vi "Climbing.vi"(0 "Start Climb?":bool) -> ()   [LabVIEW 2018]
uses:
  <vilib>/Rock Robotics/WPI/Solenoid/WPI_SolenoidValue.ctl
  <vilib>/Rock Robotics/WPI/Utilities/WPI_GetSetVariantRefNum.vi
  Robot Global Data.vi
  <vilib>/Rock Robotics/WPI/Solenoid/WPI_SolenoidSetEnum.vi
  <vilib>/Rock Robotics/WPI/RobotDrive/WPI_RobotDriveArcadeDrive_Standard(NoSaturation).vi
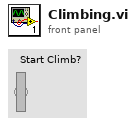
[diagram p1: front panel]
types:
  T1 = typedef "WPI_SolenoidValue.ctl" = enum16{"Off", "On", "Forward", "Reverse"}
  T2 = typedef "WPI_SolenoidDevRef.ctl" = cluster{"DevStatus":errorcluster, "Pneumatics Control Module":u8, "Forward Solenoid Channel":T3, "Reverse Solenoid Channel":T3}
  T3 = typedef "WPI_SolenoidChannel.ctl" = enum8{"Solenoid 0", "Solenoid 1", "Solenoid 2", "Solenoid 3", "Solenoid 4", "Solenoid 5", "Solenoid 6", "Solenoid 7", "Invalid"}
  T4 = typedef "WPI_RobotDriveDevRef.ctl" = cluster{"DevStatus":errorcluster, "Motors[]":T5[], "Square Inputs":bool, "Max Output":dbl}
  T5 = typedef "WPI_MotorControlDeviceRef.ctl" = cluster{"DeviceStatus":errorcluster, "Type":T6, "PWM":cluster{"PWM Channel":T7, "DeadBand":T8}, "CAN":cluster{"Device Number":u8, "SetOutput VI Ref":variant, "GetOutput VI Ref":variant, "Enable VI Ref":variant, "Disable VI Ref":variant, "Data":variant}, "Invert":bool, "DIO PWM":cluster{"PWM \"Enable\" Channel":T7, "DIOChannel":T9, "PWM Rate":dbl}}
  T6 = typedef "WPI_MotorControlType.ctl" = enum16{"PWM", "CAN", "DIO PWM"}
  T7 = typedef "FPGA_DIOPWMChannel.ctl" = enum8{"PWM 0", "PWM 1", "PWM 2", "PWM 3", "PWM 4", "PWM 5", "PWM 6", "PWM 7", "PWM 8", "PWM 9", "PWM MXP 0", "PWM MXP 1", "PWM MXP 2", "PWM MXP 3", "PWM MXP 4", "PWM MXP 5", "PWM MXP 6", "PWM MXP 7", "PWM MXP 8", "PWM MXP 9", "Invalid"}
  T8 = typedef "WPI_PWMDeadband.ctl" = cluster{"Name":string, "maxPositivePwm":i32, "minPositivePwm":i32, "centerPwm":i32, "maxNegativePwm":i32, "minNegativePwm":i32, "angularRange":u16}
  T9 = typedef "FPGA_DIOChannel.ctl" = enum8{"DIO 0", "DIO 1", "DIO 2", "DIO 3", "DIO 4", "DIO 5", "DIO 6", "DIO 7", "DIO 8", "DIO 9", "DIO MXP 0", "DIO MXP 1", "DIO MXP 2", "DIO MXP 3", "DIO MXP 4", "DIO MXP 5", "DIO MXP 6", "DIO MXP 7", "DIO MXP 8", "DIO MXP 9", "DIO MXP 10", "DIO MXP 11", "DIO MXP 12", "DIO MXP 13", "DIO MXP 14", "DIO MXP 15", "SPI Port CS1", "SPI Port CS2", "SPI Port CS3", "SPI Port MISO", "SPI Port MOSI", "Invalid"}
  T10 = typedef "WPI_DigitalInputDevRef.ctl" = cluster{"DevStatus":errorcluster, "DIO Channel":T9}
  T11 = cluster{"X-Axis":dbl, "Y-Axis":dbl, "Z-Axis":dbl}
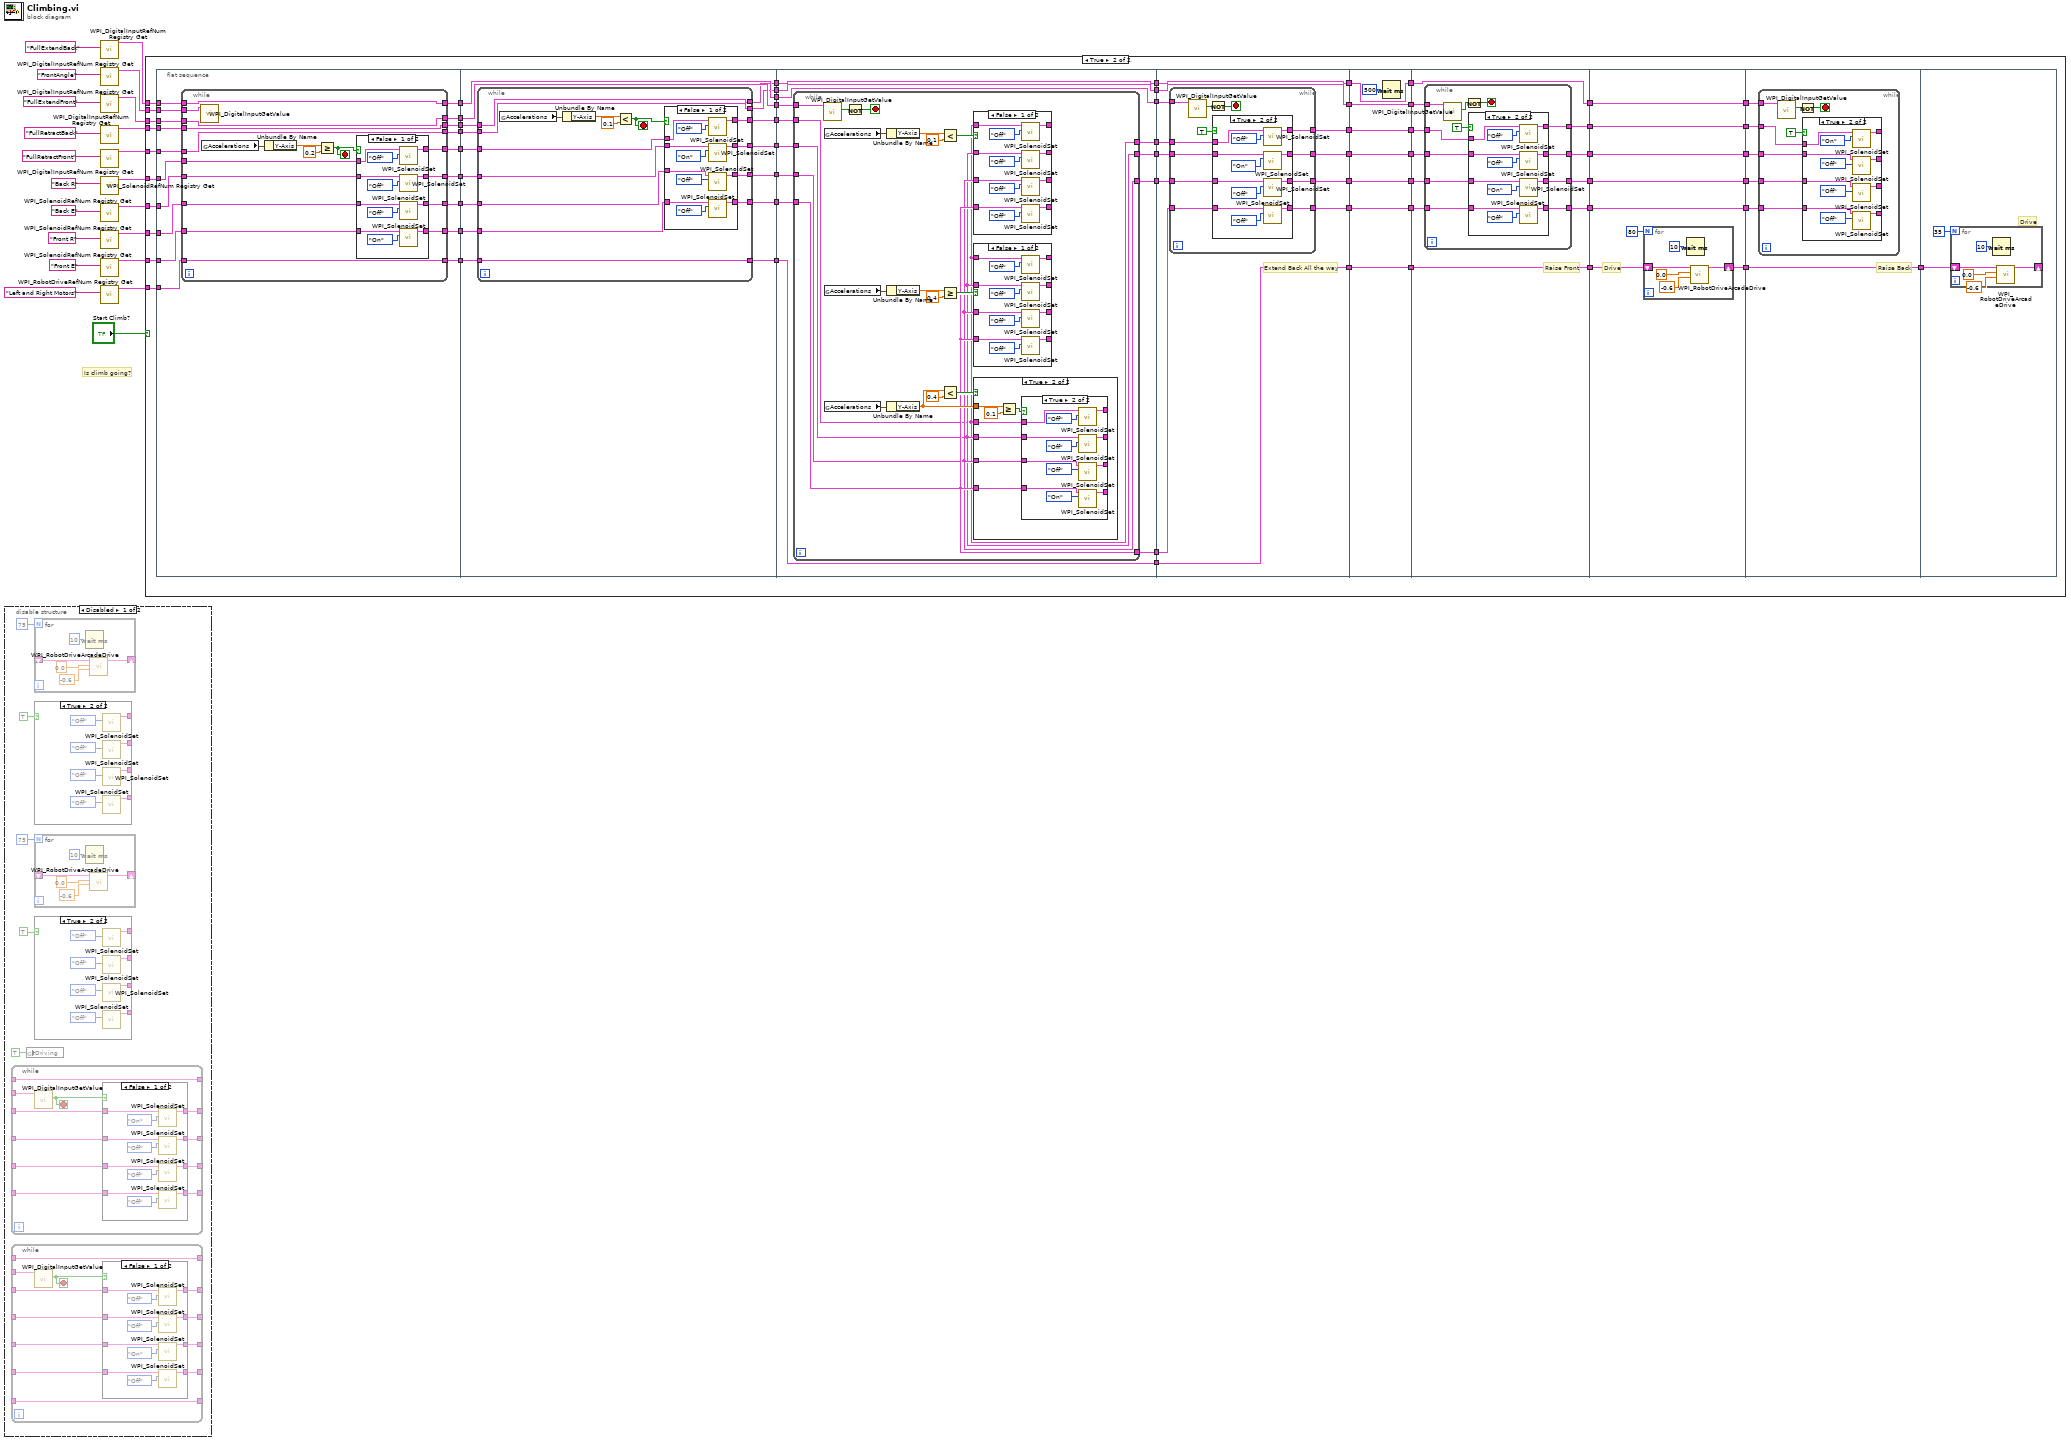
[diagram p0: block diagram]
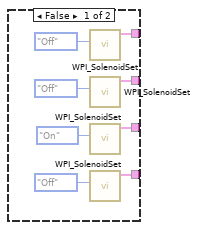
[diagram p2: hidden frame]
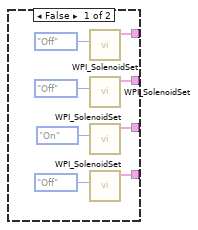
[diagram p3: hidden frame]
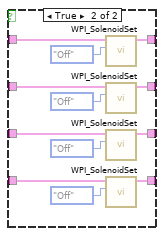
[diagram p4: hidden frame]
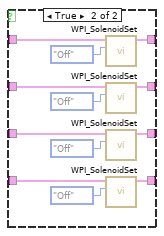
[diagram p5: hidden frame]
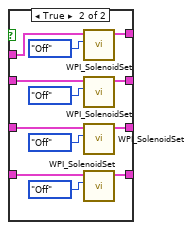
[diagram p8: hidden frame]
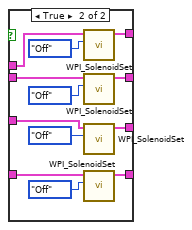
[diagram p9: hidden frame]
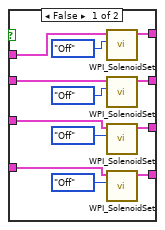
[diagram p11: hidden frame]
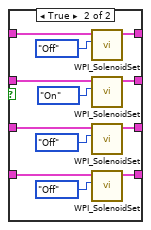
[diagram p12: hidden frame]
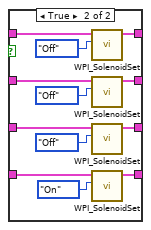
[diagram p13: hidden frame]
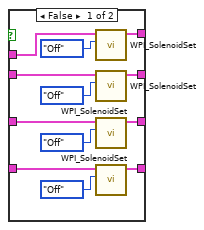
[diagram p14: hidden frame]
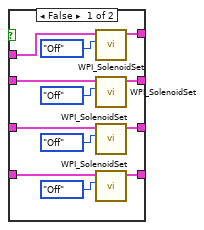
[diagram p15: hidden frame]
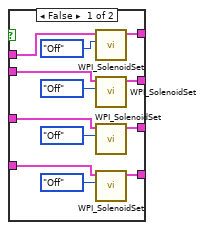
[diagram p16: hidden frame]
diagram:
  # "Is climb going?"
  n1 = disable-structure shown="Disabled" {
    frame Disabled {
      n2 = while {
        tunnel: _ -> [w79]
        tunnel: _ -> [w78]
        tunnel: _ -> [w77]
        tunnel: _ -> [w76]
        tunnel: [w75] -> _
        tunnel: _ -> [w75]
        tunnel: _ -> [w74]
        tunnel: [w72] -> _
        tunnel: [w71] -> _
        tunnel: [w70] -> _
        tunnel: [w69] -> _
        stop <- w73 stop-if-true
        n3 = call <vilib>:"WPI_DigitalInputGetValue.vi"("DigitalInputDevRef"=w74) -> ("Value"=w73:bool)  [unwired: 8 in, 2 out]
        n4 = case shown="False" w73 {
          tunnel: w76 -> [w87 w96]
          tunnel: w77 -> [w86 w97]
          tunnel: w78 -> [w85 w98]
          tunnel: w79 -> [w84 w99]
          tunnel: [w83 w95] -> w69
          tunnel: [w82 w94] -> w70
          tunnel: [w81 w93] -> w71
          tunnel: [w80 w92] -> w72
          frame False {
            n5 = call-poly <vilib>:"WPI_SolenoidSet.vi"("Value"=WPI_SolenoidValue."On", "SolenoidDevRef"=w84) -> ("SolenoidDevRef"=w80:T2)  [unwired: 8 in, 1 out]
            n6 = call-poly <vilib>:"WPI_SolenoidSet.vi"("Value"=WPI_SolenoidValue."Off", "SolenoidDevRef"=w85) -> ("SolenoidDevRef"=w81:T2)  [unwired: 8 in, 1 out]
            n7 = call-poly <vilib>:"WPI_SolenoidSet.vi"("Value"=WPI_SolenoidValue."Off", "SolenoidDevRef"=w86) -> ("SolenoidDevRef"=w82:T2)  [unwired: 8 in, 1 out]
            n8 = call-poly <vilib>:"WPI_SolenoidSet.vi"("Value"=WPI_SolenoidValue."Off", "SolenoidDevRef"=w87) -> ("SolenoidDevRef"=w83:T2)  [unwired: 8 in, 1 out]
          }
          frame True {
            n9 = call-poly <vilib>:"WPI_SolenoidSet.vi"("Value"=WPI_SolenoidValue."Off", "SolenoidDevRef"=w99) -> ("SolenoidDevRef"=w92:T2)  [unwired: 8 in, 1 out]
            n10 = call-poly <vilib>:"WPI_SolenoidSet.vi"("Value"=WPI_SolenoidValue."Off", "SolenoidDevRef"=w98) -> ("SolenoidDevRef"=w93:T2)  [unwired: 8 in, 1 out]
            n11 = call-poly <vilib>:"WPI_SolenoidSet.vi"("Value"=WPI_SolenoidValue."Off", "SolenoidDevRef"=w97) -> ("SolenoidDevRef"=w94:T2)  [unwired: 8 in, 1 out]
            n12 = call-poly <vilib>:"WPI_SolenoidSet.vi"("Value"=WPI_SolenoidValue."Off", "SolenoidDevRef"=w96) -> ("SolenoidDevRef"=w95:T2)  [unwired: 8 in, 1 out]
          }
        }
      }
      n13 = while {
        tunnel: _ -> [w115]
        tunnel: _ -> [w114]
        tunnel: _ -> [w113]
        tunnel: _ -> [w112]
        tunnel: _ -> [w111]
        tunnel: [w110] -> _
        tunnel: _ -> [w110]
        tunnel: [w109] -> _
        tunnel: _ -> [w109]
        tunnel: [w108] -> _
        tunnel: [w107] -> _
        tunnel: [w106] -> _
        tunnel: [w105] -> _
        stop <- w104 stop-if-true
        n14 = call <vilib>:"WPI_DigitalInputGetValue.vi"("DigitalInputDevRef"=w111) -> ("Value"=w104:bool)  [unwired: 8 in, 2 out]
        n15 = case shown="False" w104 {
          tunnel: w115 -> [w123 w132]
          tunnel: w114 -> [w122 w133]
          tunnel: w113 -> [w121 w134]
          tunnel: w112 -> [w120 w135]
          tunnel: [w119 w131] -> w105
          tunnel: [w118 w130] -> w106
          tunnel: [w117 w129] -> w107
          tunnel: [w116 w128] -> w108
          frame False {
            n16 = call-poly <vilib>:"WPI_SolenoidSet.vi"("Value"=WPI_SolenoidValue."Off", "SolenoidDevRef"=w120) -> ("SolenoidDevRef"=w116:T2)  [unwired: 8 in, 1 out]
            n17 = call-poly <vilib>:"WPI_SolenoidSet.vi"("Value"=WPI_SolenoidValue."Off", "SolenoidDevRef"=w121) -> ("SolenoidDevRef"=w117:T2)  [unwired: 8 in, 1 out]
            n18 = call-poly <vilib>:"WPI_SolenoidSet.vi"("Value"=WPI_SolenoidValue."On", "SolenoidDevRef"=w122) -> ("SolenoidDevRef"=w118:T2)  [unwired: 8 in, 1 out]
            n19 = call-poly <vilib>:"WPI_SolenoidSet.vi"("Value"=WPI_SolenoidValue."Off", "SolenoidDevRef"=w123) -> ("SolenoidDevRef"=w119:T2)  [unwired: 8 in, 1 out]
          }
          frame True {
            n20 = call-poly <vilib>:"WPI_SolenoidSet.vi"("Value"=WPI_SolenoidValue."Off", "SolenoidDevRef"=w135) -> ("SolenoidDevRef"=w128:T2)  [unwired: 8 in, 1 out]
            n21 = call-poly <vilib>:"WPI_SolenoidSet.vi"("Value"=WPI_SolenoidValue."Off", "SolenoidDevRef"=w134) -> ("SolenoidDevRef"=w129:T2)  [unwired: 8 in, 1 out]
            n22 = call-poly <vilib>:"WPI_SolenoidSet.vi"("Value"=WPI_SolenoidValue."Off", "SolenoidDevRef"=w133) -> ("SolenoidDevRef"=w130:T2)  [unwired: 8 in, 1 out]
            n23 = call-poly <vilib>:"WPI_SolenoidSet.vi"("Value"=WPI_SolenoidValue."Off", "SolenoidDevRef"=w132) -> ("SolenoidDevRef"=w131:T2)  [unwired: 8 in, 1 out]
          }
        }
      }
      n24 = global write "Robot Global Data.vi" "Driving"(TRUE ("Enable Vision")) -> ()
      n25 = for {
        N: 75 -> [_]
        shift-right: [w47] -> _
        shift-left: _ -> [w46]
        n26 = Wait (ms)(milliseconds to wait=u32 10) -> ()  [unwired: 1 out]
        n27 = call-poly <vilib>:"WPI_RobotDriveArcadeDrive.vi"("Y axis value"=-0.6, "X axis value"=0.0, "RobotDriveDevRef"=w46) -> ("RobotDriveDevRef"=w47:T4)  [unwired: 6 in, 2 out]
      }
      n28 = case shown="True" TRUE {
        tunnel: [w30 w38] -> _
        tunnel: [w29 w37] -> _
        tunnel: [w28 w36] -> _
        tunnel: [w27 w35] -> _
        frame False {
          n29 = call-poly <vilib>:"WPI_SolenoidSet.vi"("Value"=WPI_SolenoidValue."Off") -> ("SolenoidDevRef"=w27:T2)  [unwired: 9 in, 1 out]
          n30 = call-poly <vilib>:"WPI_SolenoidSet.vi"("Value"=WPI_SolenoidValue."Off") -> ("SolenoidDevRef"=w28:T2)  [unwired: 9 in, 1 out]
          n31 = call-poly <vilib>:"WPI_SolenoidSet.vi"("Value"=WPI_SolenoidValue."On") -> ("SolenoidDevRef"=w29:T2)  [unwired: 9 in, 1 out]
          n32 = call-poly <vilib>:"WPI_SolenoidSet.vi"("Value"=WPI_SolenoidValue."Off") -> ("SolenoidDevRef"=w30:T2)  [unwired: 9 in, 1 out]
        }
        frame True {
          n33 = call-poly <vilib>:"WPI_SolenoidSet.vi"("Value"=WPI_SolenoidValue."Off") -> ("SolenoidDevRef"=w35:T2)  [unwired: 9 in, 1 out]
          n34 = call-poly <vilib>:"WPI_SolenoidSet.vi"("Value"=WPI_SolenoidValue."Off") -> ("SolenoidDevRef"=w36:T2)  [unwired: 9 in, 1 out]
          n35 = call-poly <vilib>:"WPI_SolenoidSet.vi"("Value"=WPI_SolenoidValue."Off") -> ("SolenoidDevRef"=w37:T2)  [unwired: 9 in, 1 out]
          n36 = call-poly <vilib>:"WPI_SolenoidSet.vi"("Value"=WPI_SolenoidValue."Off") -> ("SolenoidDevRef"=w38:T2)  [unwired: 9 in, 1 out]
        }
      }
      n37 = for {
        N: 75 -> [_]
        shift-right: [w68] -> _
        shift-left: _ -> [w67]
        n38 = Wait (ms)(milliseconds to wait=u32 10) -> ()  [unwired: 1 out]
        n39 = call-poly <vilib>:"WPI_RobotDriveArcadeDrive.vi"("Y axis value"=-0.6, "X axis value"=0.0, "RobotDriveDevRef"=w67) -> ("RobotDriveDevRef"=w68:T4)  [unwired: 6 in, 2 out]
      }
      n40 = case shown="True" TRUE {
        tunnel: [w51 w59] -> _
        tunnel: [w50 w58] -> _
        tunnel: [w49 w57] -> _
        tunnel: [w48 w56] -> _
        frame False {
          n41 = call-poly <vilib>:"WPI_SolenoidSet.vi"("Value"=WPI_SolenoidValue."Off") -> ("SolenoidDevRef"=w48:T2)  [unwired: 9 in, 1 out]
          n42 = call-poly <vilib>:"WPI_SolenoidSet.vi"("Value"=WPI_SolenoidValue."Off") -> ("SolenoidDevRef"=w49:T2)  [unwired: 9 in, 1 out]
          n43 = call-poly <vilib>:"WPI_SolenoidSet.vi"("Value"=WPI_SolenoidValue."On") -> ("SolenoidDevRef"=w50:T2)  [unwired: 9 in, 1 out]
          n44 = call-poly <vilib>:"WPI_SolenoidSet.vi"("Value"=WPI_SolenoidValue."Off") -> ("SolenoidDevRef"=w51:T2)  [unwired: 9 in, 1 out]
        }
        frame True {
          n45 = call-poly <vilib>:"WPI_SolenoidSet.vi"("Value"=WPI_SolenoidValue."Off") -> ("SolenoidDevRef"=w56:T2)  [unwired: 9 in, 1 out]
          n46 = call-poly <vilib>:"WPI_SolenoidSet.vi"("Value"=WPI_SolenoidValue."Off") -> ("SolenoidDevRef"=w57:T2)  [unwired: 9 in, 1 out]
          n47 = call-poly <vilib>:"WPI_SolenoidSet.vi"("Value"=WPI_SolenoidValue."Off") -> ("SolenoidDevRef"=w58:T2)  [unwired: 9 in, 1 out]
          n48 = call-poly <vilib>:"WPI_SolenoidSet.vi"("Value"=WPI_SolenoidValue."Off") -> ("SolenoidDevRef"=w59:T2)  [unwired: 9 in, 1 out]
        }
      }
    }
    frame Enabled {
    }
  }
  n49 = call <vilib>:"WPI_DigitalInputRefNum Registry Get.vi"("refnum name"="FullExtendBack") -> ("DigitalInputDevRef"=w1:T10)  [unwired: 9 in, 1 out]
  n50 = call <vilib>:"WPI_DigitalInputRefNum Registry Get.vi"("refnum name"="FrontAngle") -> ("DigitalInputDevRef"=w7:T10)  [unwired: 9 in, 1 out]
  n51 = call <vilib>:"WPI_DigitalInputRefNum Registry Get.vi"("refnum name"="FullExtendFront") -> ("DigitalInputDevRef"=w9:T10)  [unwired: 9 in, 1 out]
  n52 = call <vilib>:"WPI_DigitalInputRefNum Registry Get.vi"("refnum name"="FullRetractBack") -> ("DigitalInputDevRef"=w5:T10)  [unwired: 9 in, 1 out]
  n53 = call <vilib>:"WPI_DigitalInputRefNum Registry Get.vi"("refnum name"="FullRetractFront") -> ("DigitalInputDevRef"=w3:T10)  [unwired: 9 in, 1 out]
  n54 = call <vilib>:"WPI_SolenoidRefNum Registry Get.vi"("refnum name"="Back R") -> ("SolenoidDevRef"=w13:T2)  [unwired: 9 in, 1 out]
  n55 = call <vilib>:"WPI_SolenoidRefNum Registry Get.vi"("refnum name"="Back E") -> ("SolenoidDevRef"=w15:T2)  [unwired: 9 in, 1 out]
  n56 = call <vilib>:"WPI_SolenoidRefNum Registry Get.vi"("refnum name"="Front R") -> ("SolenoidDevRef"=w14:T2)  [unwired: 9 in, 1 out]
  n57 = call <vilib>:"WPI_SolenoidRefNum Registry Get.vi"("refnum name"="Front E") -> ("SolenoidDevRef"=w16:T2)  [unwired: 9 in, 1 out]
  n58 = call <vilib>:"WPI_RobotDriveRefNum Registry Get.vi"("refnum name"="Left and Right Motors") -> ("RobotDriveDevRef"=w11:T4)  [unwired: 9 in, 1 out]
  n59 = case shown="True" "Start Climb?" {
    tunnel: w16 -> [_ w202]
    tunnel: w15 -> [_ w200]
    tunnel: w14 -> [_ w201]
    tunnel: w13 -> [_ w199]
    tunnel: w11 -> [_ w198]
    tunnel: w9 -> [_ w196]
    tunnel: w7 -> [_ w197]
    tunnel: w5 -> [_ w193]
    tunnel: w3 -> [_ w194]
    tunnel: w1 -> [_ w195]
    frame False {
    }
    frame True {
      n60 = flat-sequence {
        tunnel: w202 -> [w212]
        tunnel: w201 -> [w213]
        tunnel: w200 -> [w214]
        tunnel: w199 -> [w215]
        tunnel: w198 -> [w219]
        tunnel: w197 -> [w216]
        tunnel: w196 -> [w217]
        tunnel: w195 -> [w218]
        tunnel: w194 -> [w221]
        tunnel: w193 -> [w220]
        tunnel: [w211] -> w192
        tunnel: [w210] -> w191
        tunnel: [w209] -> w190
        tunnel: [w208] -> w189
        tunnel: [w207] -> w188
        tunnel: [w206] -> w187
        tunnel: [w205] -> w186
        tunnel: [w204] -> w180
        tunnel: [w203] -> w177
        tunnel: w192 -> [w279]
        tunnel: w191 -> [w278]
        tunnel: w190 -> [w277]
        tunnel: w189 -> [w276]
        tunnel: w188 -> [w275]
        tunnel: w187 -> [w274]
        tunnel: w186 -> [w273]
        tunnel: [w272] -> w185
        tunnel: [w271] -> w184
        tunnel: [w270] -> w183
        tunnel: [w269] -> w182
        tunnel: [w268] -> w181
        tunnel: w180 -> [w268]
        tunnel: [w267] -> w178
        tunnel: w177 -> [w267]
        tunnel: [w266] -> w171
        tunnel: [w265] -> w156
        tunnel: [w264] -> w142
        tunnel: w185 -> [w331]
        tunnel: w184 -> [w330]
        tunnel: w183 -> [w329]
        tunnel: w182 -> [w328]
        tunnel: w181 -> [w327]
        tunnel: [w326] -> w179
        tunnel: w178 -> [w326]
        tunnel: [w325] -> w176
        tunnel: [w324] -> w175
        tunnel: [w323] -> w174
        tunnel: [w322] -> w173
        tunnel: [w321] -> w172
        tunnel: w171 -> [w321]
        tunnel: [w320] -> w157
        tunnel: w156 -> [w320]
        tunnel: [w319] -> w143
        tunnel: w142 -> [w319]
        tunnel: w179 -> [w441]
        tunnel: w176 -> [w440]
        tunnel: w175 -> [w439]
        tunnel: w174 -> [w438]
        tunnel: w173 -> [w437]
        tunnel: [w436] -> w170
        tunnel: w172 -> [w436]
        tunnel: [w435] -> w168
        tunnel: [w434] -> w166
        tunnel: [w433] -> w164
        tunnel: [w432] -> w162
        tunnel: [w431] -> w158
        tunnel: w157 -> [w431]
        tunnel: [w430] -> w144
        tunnel: w143 -> [w430]
        tunnel: w170 -> [w485]
        tunnel: [w485] -> w169
        tunnel: w168 -> [w484]
        tunnel: [w484] -> w167
        tunnel: w166 -> [w483]
        tunnel: [w483] -> w165
        tunnel: w164 -> [w482]
        tunnel: [w482] -> w163
        tunnel: w162 -> [w481]
        tunnel: [w481] -> w161
        tunnel: [w479] -> w159
        tunnel: w158 -> [w479]
        tunnel: [w478] -> w145
        tunnel: w144 -> [w478]
        tunnel: w169 -> [w496]
        tunnel: w167 -> [w495]
        tunnel: w165 -> [w494]
        tunnel: w163 -> [w493]
        tunnel: w161 -> [w492]
        tunnel: [w491] -> w160
        tunnel: w159 -> [w491]
        tunnel: [w490] -> w155
        tunnel: [w489] -> w152
        tunnel: [w488] -> w150
        tunnel: [w487] -> w148
        tunnel: [w486] -> w146
        tunnel: w145 -> [w486]
        tunnel: w160 -> [w539]
        tunnel: w155 -> [w538]
        tunnel: [w538] -> w154
        tunnel: [w537] -> w153
        tunnel: w152 -> [w537]
        tunnel: [w536] -> w151
        tunnel: w150 -> [w536]
        tunnel: [w535] -> w149
        tunnel: w148 -> [w535]
        tunnel: [w534] -> w147
        tunnel: w146 -> [w534]
        tunnel: [w533] -> w140
        tunnel: w154 -> [w551]
        tunnel: w153 -> [w550]
        tunnel: w151 -> [w549]
        tunnel: w149 -> [w548]
        tunnel: w147 -> [w547]
        tunnel: [w546] -> w141
        tunnel: w140 -> [w546]
        tunnel: w141 -> [w584]
        frame #0 {
          n61 = while {
            tunnel: w212 -> [w239]
            tunnel: w213 -> [w238]
            tunnel: w214 -> [w237]
            tunnel: w215 -> [w236]
            tunnel: [w235] -> w206
            tunnel: [w234] -> w205
            tunnel: [w233] -> w207
            tunnel: [w232] -> w208
            tunnel: [w231] -> w209
            tunnel: w219 -> [w231]
            tunnel: w216 -> [w230]
            tunnel: [w229] -> w204
            tunnel: w217 -> [w229]
            tunnel: [w228] -> w203
            tunnel: w218 -> [w228]
            tunnel: [w227] -> w211
            tunnel: w221 -> [w227]
            tunnel: [w226] -> w210
            tunnel: w220 -> [w226]
            stop <- w222 stop-if-true
            n62 = call <vilib>:"WPI_DigitalInputGetValue.vi"("DigitalInputDevRef"=w230) -> ()  [unwired: 8 in, 3 out]
            n63 = global read "Robot Global Data.vi" "Accelerations"() -> (w225:T11)
            n64 = Unbundle By Name(w225) -> ("Y-Axis"=w224:dbl)
            n65 = Greater Or Equal?(x=w224, y=0.2) -> (x >= y?=w222:bool)
            n66 = case shown="False" w222 {
              tunnel: w239 -> [w247 w256]
              tunnel: w238 -> [w246 w257]
              tunnel: w237 -> [w245 w258]
              tunnel: w236 -> [w244 w259]
              tunnel: [w243 w252] -> w234
              tunnel: [w242 w253] -> w235
              tunnel: [w241 w254] -> w233
              tunnel: [w240 w255] -> w232
              frame False {
                n67 = call-poly <vilib>:"WPI_SolenoidSet.vi"("Value"=WPI_SolenoidValue."Off", "SolenoidDevRef"=w244) -> ("SolenoidDevRef"=w240:T2)  [unwired: 8 in, 1 out]
                n68 = call-poly <vilib>:"WPI_SolenoidSet.vi"("Value"=WPI_SolenoidValue."Off", "SolenoidDevRef"=w245) -> ("SolenoidDevRef"=w241:T2)  [unwired: 8 in, 1 out]
                n69 = call-poly <vilib>:"WPI_SolenoidSet.vi"("Value"=WPI_SolenoidValue."Off", "SolenoidDevRef"=w246) -> ("SolenoidDevRef"=w242:T2)  [unwired: 8 in, 1 out]
                n70 = call-poly <vilib>:"WPI_SolenoidSet.vi"("Value"=WPI_SolenoidValue."On", "SolenoidDevRef"=w247) -> ("SolenoidDevRef"=w243:T2)  [unwired: 8 in, 1 out]
              }
              frame True {
                n71 = call-poly <vilib>:"WPI_SolenoidSet.vi"("Value"=WPI_SolenoidValue."Off", "SolenoidDevRef"=w259) -> ("SolenoidDevRef"=w255:T2)  [unwired: 8 in, 1 out]
                n72 = call-poly <vilib>:"WPI_SolenoidSet.vi"("Value"=WPI_SolenoidValue."Off", "SolenoidDevRef"=w258) -> ("SolenoidDevRef"=w254:T2)  [unwired: 8 in, 1 out]
                n73 = call-poly <vilib>:"WPI_SolenoidSet.vi"("Value"=WPI_SolenoidValue."Off", "SolenoidDevRef"=w257) -> ("SolenoidDevRef"=w253:T2)  [unwired: 8 in, 1 out]
                n74 = call-poly <vilib>:"WPI_SolenoidSet.vi"("Value"=WPI_SolenoidValue."Off", "SolenoidDevRef"=w256) -> ("SolenoidDevRef"=w252:T2)  [unwired: 8 in, 1 out]
              }
            }
          }
        }
        frame #1 {
          n75 = while {
            tunnel: w276 -> [w294]
            tunnel: w275 -> [w293]
            tunnel: w274 -> [w292]
            tunnel: w273 -> [w291]
            tunnel: [w290] -> w265
            tunnel: w277 -> [w290]
            tunnel: [w289] -> w272
            tunnel: [w288] -> w271
            tunnel: [w287] -> w270
            tunnel: [w286] -> w269
            tunnel: [w282] -> w266
            tunnel: w279 -> [w282]
            tunnel: [w281] -> w264
            tunnel: w278 -> [w281]
            stop <- w280 stop-if-true
            n76 = global read "Robot Global Data.vi" "Accelerations"() -> (w285:T11)
            n77 = Unbundle By Name(w285) -> ("Y-Axis"=w284:dbl)
            n78 = Less?(x=w284, y=0.1) -> (x < y?=w280:bool)
            n79 = case shown="False" w280 {
              tunnel: w291 -> [w302 w311]
              tunnel: w292 -> [w301 w312]
              tunnel: w293 -> [w300 w313]
              tunnel: w294 -> [w299 w314]
              tunnel: [w298 w310] -> w286
              tunnel: [w297 w309] -> w287
              tunnel: [w296 w308] -> w288
              tunnel: [w295 w307] -> w289
              frame False {
                n80 = call-poly <vilib>:"WPI_SolenoidSet.vi"("Value"=WPI_SolenoidValue."Off", "SolenoidDevRef"=w299) -> ("SolenoidDevRef"=w295:T2)  [unwired: 8 in, 1 out]
                n81 = call-poly <vilib>:"WPI_SolenoidSet.vi"("Value"=WPI_SolenoidValue."On", "SolenoidDevRef"=w300) -> ("SolenoidDevRef"=w296:T2)  [unwired: 8 in, 1 out]
                n82 = call-poly <vilib>:"WPI_SolenoidSet.vi"("Value"=WPI_SolenoidValue."Off", "SolenoidDevRef"=w301) -> ("SolenoidDevRef"=w297:T2)  [unwired: 8 in, 1 out]
                n83 = call-poly <vilib>:"WPI_SolenoidSet.vi"("Value"=WPI_SolenoidValue."Off", "SolenoidDevRef"=w302) -> ("SolenoidDevRef"=w298:T2)  [unwired: 8 in, 1 out]
              }
              frame True {
                n84 = call-poly <vilib>:"WPI_SolenoidSet.vi"("Value"=WPI_SolenoidValue."Off", "SolenoidDevRef"=w314) -> ("SolenoidDevRef"=w307:T2)  [unwired: 8 in, 1 out]
                n85 = call-poly <vilib>:"WPI_SolenoidSet.vi"("Value"=WPI_SolenoidValue."Off", "SolenoidDevRef"=w313) -> ("SolenoidDevRef"=w308:T2)  [unwired: 8 in, 1 out]
                n86 = call-poly <vilib>:"WPI_SolenoidSet.vi"("Value"=WPI_SolenoidValue."Off", "SolenoidDevRef"=w312) -> ("SolenoidDevRef"=w309:T2)  [unwired: 8 in, 1 out]
                n87 = call-poly <vilib>:"WPI_SolenoidSet.vi"("Value"=WPI_SolenoidValue."Off", "SolenoidDevRef"=w311) -> ("SolenoidDevRef"=w310:T2)  [unwired: 8 in, 1 out]
              }
            }
          }
        }
        frame #2 {
          n88 = while {
            tunnel: w331 -> [w332]
            tunnel: w330 -> [w333]
            tunnel: w329 -> [w334]
            tunnel: w328 -> [w335]
            tunnel: w327 -> [w342]
            tunnel: [w335] -> w325
            tunnel: [w334] -> w324
            tunnel: [w333] -> w323
            tunnel: [w332] -> w322
            stop <- w340 stop-if-true
            n89 = call <vilib>:"WPI_DigitalInputGetValue.vi"("DigitalInputDevRef"=w342) -> ("Value"=w341:bool)  [unwired: 8 in, 2 out]
            n90 = global read "Robot Global Data.vi" "Accelerations"() -> (w348:T11)
            n91 = global read "Robot Global Data.vi" "Accelerations"() -> (w344:T11)
            n92 = global read "Robot Global Data.vi" "Accelerations"() -> (w338:T11)
            n93 = Not(x=w341) -> (.not. x?=w340:bool)
            n94 = Unbundle By Name(w348) -> ("Y-Axis"=w349:dbl)
            n95 = Unbundle By Name(w344) -> ("Y-Axis"=w345:dbl)
            n96 = Unbundle By Name(w338) -> ("Y-Axis"=w337:dbl)
            n97 = Less?(x=w349, y=0.1) -> (x < y?=w347:bool)
            n98 = Greater Or Equal?(x=w345, y=0.4) -> (x >= y?=w343:bool)
            n99 = Less?(x=w337, y=0.4) -> (x < y?=w339:bool)
            n100 = case shown="False" w347 {
              tunnel: w335 -> [w413 w422]
              tunnel: w334 -> [w412 w423]
              tunnel: w333 -> [w411 w424]
              tunnel: w332 -> [w410 w425]
              tunnel: [w409 w421] -> _
              tunnel: [w408 w420] -> _
              tunnel: [w407 w419] -> _
              tunnel: [w406 w418] -> _
              frame False {
                n101 = call-poly <vilib>:"WPI_SolenoidSet.vi"("Value"=WPI_SolenoidValue."Off", "SolenoidDevRef"=w410) -> ("SolenoidDevRef"=w406:T2)  [unwired: 8 in, 1 out]
                n102 = call-poly <vilib>:"WPI_SolenoidSet.vi"("Value"=WPI_SolenoidValue."Off", "SolenoidDevRef"=w411) -> ("SolenoidDevRef"=w407:T2)  [unwired: 8 in, 1 out]
                n103 = call-poly <vilib>:"WPI_SolenoidSet.vi"("Value"=WPI_SolenoidValue."Off", "SolenoidDevRef"=w412) -> ("SolenoidDevRef"=w408:T2)  [unwired: 8 in, 1 out]
                n104 = call-poly <vilib>:"WPI_SolenoidSet.vi"("Value"=WPI_SolenoidValue."Off", "SolenoidDevRef"=w413) -> ("SolenoidDevRef"=w409:T2)  [unwired: 8 in, 1 out]
              }
              frame True {
                n105 = call-poly <vilib>:"WPI_SolenoidSet.vi"("Value"=WPI_SolenoidValue."Off", "SolenoidDevRef"=w425) -> ("SolenoidDevRef"=w418:T2)  [unwired: 8 in, 1 out]
                n106 = call-poly <vilib>:"WPI_SolenoidSet.vi"("Value"=WPI_SolenoidValue."Off", "SolenoidDevRef"=w424) -> ("SolenoidDevRef"=w419:T2)  [unwired: 8 in, 1 out]
                n107 = call-poly <vilib>:"WPI_SolenoidSet.vi"("Value"=WPI_SolenoidValue."Off", "SolenoidDevRef"=w423) -> ("SolenoidDevRef"=w420:T2)  [unwired: 8 in, 1 out]
                n108 = call-poly <vilib>:"WPI_SolenoidSet.vi"("Value"=WPI_SolenoidValue."On", "SolenoidDevRef"=w422) -> ("SolenoidDevRef"=w421:T2)  [unwired: 8 in, 1 out]
              }
            }
            n109 = case shown="False" w343 {
              tunnel: w335 -> [w389 w398]
              tunnel: w334 -> [w388 w399]
              tunnel: w333 -> [w387 w400]
              tunnel: w332 -> [w386 w401]
              tunnel: [w385 w397] -> _
              tunnel: [w384 w396] -> _
              tunnel: [w383 w395] -> _
              tunnel: [w382 w394] -> _
              frame False {
                n110 = call-poly <vilib>:"WPI_SolenoidSet.vi"("Value"=WPI_SolenoidValue."Off", "SolenoidDevRef"=w386) -> ("SolenoidDevRef"=w382:T2)  [unwired: 8 in, 1 out]
                n111 = call-poly <vilib>:"WPI_SolenoidSet.vi"("Value"=WPI_SolenoidValue."Off", "SolenoidDevRef"=w387) -> ("SolenoidDevRef"=w383:T2)  [unwired: 8 in, 1 out]
                n112 = call-poly <vilib>:"WPI_SolenoidSet.vi"("Value"=WPI_SolenoidValue."Off", "SolenoidDevRef"=w388) -> ("SolenoidDevRef"=w384:T2)  [unwired: 8 in, 1 out]
                n113 = call-poly <vilib>:"WPI_SolenoidSet.vi"("Value"=WPI_SolenoidValue."Off", "SolenoidDevRef"=w389) -> ("SolenoidDevRef"=w385:T2)  [unwired: 8 in, 1 out]
              }
              frame True {
                n114 = call-poly <vilib>:"WPI_SolenoidSet.vi"("Value"=WPI_SolenoidValue."Off", "SolenoidDevRef"=w401) -> ("SolenoidDevRef"=w394:T2)  [unwired: 8 in, 1 out]
                n115 = call-poly <vilib>:"WPI_SolenoidSet.vi"("Value"=WPI_SolenoidValue."On", "SolenoidDevRef"=w400) -> ("SolenoidDevRef"=w395:T2)  [unwired: 8 in, 1 out]
                n116 = call-poly <vilib>:"WPI_SolenoidSet.vi"("Value"=WPI_SolenoidValue."Off", "SolenoidDevRef"=w399) -> ("SolenoidDevRef"=w396:T2)  [unwired: 8 in, 1 out]
                n117 = call-poly <vilib>:"WPI_SolenoidSet.vi"("Value"=WPI_SolenoidValue."Off", "SolenoidDevRef"=w398) -> ("SolenoidDevRef"=w397:T2)  [unwired: 8 in, 1 out]
              }
            }
            n118 = case shown="True" w339 {
              tunnel: w335 -> [_ w356]
              tunnel: w334 -> [_ w355]
              tunnel: w333 -> [_ w354]
              tunnel: w332 -> [_ w353]
              tunnel: w337 -> [_ w352]
              frame False {
              }
              frame True {
                n119 = Greater Or Equal?(x=w352, y=0.1) -> (x >= y?=w357:bool)
                n120 = case shown="True" w357 {
                  tunnel: w356 -> [w365 w374]
                  tunnel: w355 -> [w364 w375]
                  tunnel: w354 -> [w363 w376]
                  tunnel: w353 -> [w362 w377]
                  tunnel: [w361 w373] -> _
                  tunnel: [w360 w372] -> _
                  tunnel: [w359 w371] -> _
                  tunnel: [w358 w370] -> _
                  frame False {
                    n121 = call-poly <vilib>:"WPI_SolenoidSet.vi"("Value"=WPI_SolenoidValue."Off", "SolenoidDevRef"=w362) -> ("SolenoidDevRef"=w358:T2)  [unwired: 8 in, 1 out]
                    n122 = call-poly <vilib>:"WPI_SolenoidSet.vi"("Value"=WPI_SolenoidValue."Off", "SolenoidDevRef"=w363) -> ("SolenoidDevRef"=w359:T2)  [unwired: 8 in, 1 out]
                    n123 = call-poly <vilib>:"WPI_SolenoidSet.vi"("Value"=WPI_SolenoidValue."Off", "SolenoidDevRef"=w364) -> ("SolenoidDevRef"=w360:T2)  [unwired: 8 in, 1 out]
                    n124 = call-poly <vilib>:"WPI_SolenoidSet.vi"("Value"=WPI_SolenoidValue."Off", "SolenoidDevRef"=w365) -> ("SolenoidDevRef"=w361:T2)  [unwired: 8 in, 1 out]
                  }
                  frame True {
                    n125 = call-poly <vilib>:"WPI_SolenoidSet.vi"("Value"=WPI_SolenoidValue."Off", "SolenoidDevRef"=w377) -> ("SolenoidDevRef"=w370:T2)  [unwired: 8 in, 1 out]
                    n126 = call-poly <vilib>:"WPI_SolenoidSet.vi"("Value"=WPI_SolenoidValue."Off", "SolenoidDevRef"=w376) -> ("SolenoidDevRef"=w371:T2)  [unwired: 8 in, 1 out]
                    n127 = call-poly <vilib>:"WPI_SolenoidSet.vi"("Value"=WPI_SolenoidValue."Off", "SolenoidDevRef"=w375) -> ("SolenoidDevRef"=w372:T2)  [unwired: 8 in, 1 out]
                    n128 = call-poly <vilib>:"WPI_SolenoidSet.vi"("Value"=WPI_SolenoidValue."On", "SolenoidDevRef"=w374) -> ("SolenoidDevRef"=w373:T2)  [unwired: 8 in, 1 out]
                  }
                }
              }
            }
          }
        }
        frame #3 {
          # "Extend Back All the way"
          n129 = while {
            tunnel: w441 -> [w453]
            tunnel: w440 -> [w450]
            tunnel: w439 -> [w449]
            tunnel: w438 -> [w448]
            tunnel: w437 -> [w447]
            tunnel: [w445] -> w435
            tunnel: [w444] -> w434
            tunnel: [w443] -> w433
            tunnel: [w442] -> w432
            stop <- w451 stop-if-true
            n130 = call <vilib>:"WPI_DigitalInputGetValue.vi"("DigitalInputDevRef"=w453) -> ("Value"=w452:bool)  [unwired: 8 in, 2 out]
            n131 = Not(x=w452) -> (.not. x?=w451:bool)
            n132 = case shown="True" TRUE {
              tunnel: w450 -> [w461 w470]
              tunnel: w449 -> [w460 w471]
              tunnel: w448 -> [w459 w472]
              tunnel: w447 -> [w458 w473]
              tunnel: [w457 w469] -> w445
              tunnel: [w456 w468] -> w444
              tunnel: [w455 w467] -> w443
              tunnel: [w454 w466] -> w442
              frame False {
                n133 = call-poly <vilib>:"WPI_SolenoidSet.vi"("Value"=WPI_SolenoidValue."Off", "SolenoidDevRef"=w458) -> ("SolenoidDevRef"=w454:T2)  [unwired: 8 in, 1 out]
                n134 = call-poly <vilib>:"WPI_SolenoidSet.vi"("Value"=WPI_SolenoidValue."Off", "SolenoidDevRef"=w459) -> ("SolenoidDevRef"=w455:T2)  [unwired: 8 in, 1 out]
                n135 = call-poly <vilib>:"WPI_SolenoidSet.vi"("Value"=WPI_SolenoidValue."Off", "SolenoidDevRef"=w460) -> ("SolenoidDevRef"=w456:T2)  [unwired: 8 in, 1 out]
                n136 = call-poly <vilib>:"WPI_SolenoidSet.vi"("Value"=WPI_SolenoidValue."Off", "SolenoidDevRef"=w461) -> ("SolenoidDevRef"=w457:T2)  [unwired: 8 in, 1 out]
              }
              frame True {
                n137 = call-poly <vilib>:"WPI_SolenoidSet.vi"("Value"=WPI_SolenoidValue."Off", "SolenoidDevRef"=w473) -> ("SolenoidDevRef"=w466:T2)  [unwired: 8 in, 1 out]
                n138 = call-poly <vilib>:"WPI_SolenoidSet.vi"("Value"=WPI_SolenoidValue."On", "SolenoidDevRef"=w472) -> ("SolenoidDevRef"=w467:T2)  [unwired: 8 in, 1 out]
                n139 = call-poly <vilib>:"WPI_SolenoidSet.vi"("Value"=WPI_SolenoidValue."Off", "SolenoidDevRef"=w471) -> ("SolenoidDevRef"=w468:T2)  [unwired: 8 in, 1 out]
                n140 = call-poly <vilib>:"WPI_SolenoidSet.vi"("Value"=WPI_SolenoidValue."Off", "SolenoidDevRef"=w470) -> ("SolenoidDevRef"=w469:T2)  [unwired: 8 in, 1 out]
              }
            }
          }
        }
        frame #4 {
          n141 = Wait (ms)(milliseconds to wait=u32 500) -> ()  [unwired: 1 out]
        }
        frame #5 {
          # "Raise Front"
          n142 = while {
            tunnel: w496 -> [w508]
            tunnel: w495 -> [w504]
            tunnel: w494 -> [w503]
            tunnel: w493 -> [w502]
            tunnel: w492 -> [w501]
            tunnel: [w500] -> w490
            tunnel: [w499] -> w489
            tunnel: [w498] -> w488
            tunnel: [w497] -> w487
            stop <- w506 stop-if-true
            n143 = call <vilib>:"WPI_DigitalInputGetValue.vi"("DigitalInputDevRef"=w508) -> ("Value"=w507:bool)  [unwired: 8 in, 2 out]
            n144 = Not(x=w507) -> (.not. x?=w506:bool)
            n145 = case shown="True" TRUE {
              tunnel: w504 -> [w516 w525]
              tunnel: w503 -> [w515 w526]
              tunnel: w502 -> [w514 w527]
              tunnel: w501 -> [w513 w528]
              tunnel: [w512 w524] -> w500
              tunnel: [w511 w523] -> w499
              tunnel: [w510 w522] -> w498
              tunnel: [w509 w521] -> w497
              frame False {
                n146 = call-poly <vilib>:"WPI_SolenoidSet.vi"("Value"=WPI_SolenoidValue."Off", "SolenoidDevRef"=w513) -> ("SolenoidDevRef"=w509:T2)  [unwired: 8 in, 1 out]
                n147 = call-poly <vilib>:"WPI_SolenoidSet.vi"("Value"=WPI_SolenoidValue."Off", "SolenoidDevRef"=w514) -> ("SolenoidDevRef"=w510:T2)  [unwired: 8 in, 1 out]
                n148 = call-poly <vilib>:"WPI_SolenoidSet.vi"("Value"=WPI_SolenoidValue."Off", "SolenoidDevRef"=w515) -> ("SolenoidDevRef"=w511:T2)  [unwired: 8 in, 1 out]
                n149 = call-poly <vilib>:"WPI_SolenoidSet.vi"("Value"=WPI_SolenoidValue."Off", "SolenoidDevRef"=w516) -> ("SolenoidDevRef"=w512:T2)  [unwired: 8 in, 1 out]
              }
              frame True {
                n150 = call-poly <vilib>:"WPI_SolenoidSet.vi"("Value"=WPI_SolenoidValue."Off", "SolenoidDevRef"=w528) -> ("SolenoidDevRef"=w521:T2)  [unwired: 8 in, 1 out]
                n151 = call-poly <vilib>:"WPI_SolenoidSet.vi"("Value"=WPI_SolenoidValue."Off", "SolenoidDevRef"=w527) -> ("SolenoidDevRef"=w522:T2)  [unwired: 8 in, 1 out]
                n152 = call-poly <vilib>:"WPI_SolenoidSet.vi"("Value"=WPI_SolenoidValue."On", "SolenoidDevRef"=w526) -> ("SolenoidDevRef"=w523:T2)  [unwired: 8 in, 1 out]
                n153 = call-poly <vilib>:"WPI_SolenoidSet.vi"("Value"=WPI_SolenoidValue."Off", "SolenoidDevRef"=w525) -> ("SolenoidDevRef"=w524:T2)  [unwired: 8 in, 1 out]
              }
            }
          }
        }
        frame #6 {
          # "Drive"
          n154 = for {
            N: 80 -> [_]
            shift-right: [w545] -> w533
            shift-left: w539 -> [w544]
            n155 = Wait (ms)(milliseconds to wait=u32 10) -> ()  [unwired: 1 out]
            n156 = call-poly <vilib>:"WPI_RobotDriveArcadeDrive.vi"("Y axis value"=-0.6, "X axis value"=0.0, "RobotDriveDevRef"=w544) -> ("RobotDriveDevRef"=w545:T4)  [unwired: 6 in, 2 out]
          }
        }
        frame #7 {
          # "Raise Back"
          n157 = while {
            tunnel: w551 -> [w556]
            tunnel: w550 -> [w555]
            tunnel: w549 -> [w554]
            tunnel: w548 -> [w553]
            tunnel: w547 -> [w552]
            stop <- w558 stop-if-true
            n158 = call <vilib>:"WPI_DigitalInputGetValue.vi"("DigitalInputDevRef"=w552) -> ("Value"=w559:bool)  [unwired: 8 in, 2 out]
            n159 = Not(x=w559) -> (.not. x?=w558:bool)
            n160 = case shown="True" TRUE {
              tunnel: w556 -> [w567 w576]
              tunnel: w555 -> [w566 w577]
              tunnel: w554 -> [w565 w578]
              tunnel: w553 -> [w564 w579]
              tunnel: [w563 w575] -> _
              tunnel: [w562 w574] -> _
              tunnel: [w561 w573] -> _
              tunnel: [w560 w572] -> _
              frame False {
                n161 = call-poly <vilib>:"WPI_SolenoidSet.vi"("Value"=WPI_SolenoidValue."Off", "SolenoidDevRef"=w564) -> ("SolenoidDevRef"=w560:T2)  [unwired: 8 in, 1 out]
                n162 = call-poly <vilib>:"WPI_SolenoidSet.vi"("Value"=WPI_SolenoidValue."Off", "SolenoidDevRef"=w565) -> ("SolenoidDevRef"=w561:T2)  [unwired: 8 in, 1 out]
                n163 = call-poly <vilib>:"WPI_SolenoidSet.vi"("Value"=WPI_SolenoidValue."Off", "SolenoidDevRef"=w566) -> ("SolenoidDevRef"=w562:T2)  [unwired: 8 in, 1 out]
                n164 = call-poly <vilib>:"WPI_SolenoidSet.vi"("Value"=WPI_SolenoidValue."Off", "SolenoidDevRef"=w567) -> ("SolenoidDevRef"=w563:T2)  [unwired: 8 in, 1 out]
              }
              frame True {
                n165 = call-poly <vilib>:"WPI_SolenoidSet.vi"("Value"=WPI_SolenoidValue."On", "SolenoidDevRef"=w579) -> ("SolenoidDevRef"=w572:T2)  [unwired: 8 in, 1 out]
                n166 = call-poly <vilib>:"WPI_SolenoidSet.vi"("Value"=WPI_SolenoidValue."Off", "SolenoidDevRef"=w578) -> ("SolenoidDevRef"=w573:T2)  [unwired: 8 in, 1 out]
                n167 = call-poly <vilib>:"WPI_SolenoidSet.vi"("Value"=WPI_SolenoidValue."Off", "SolenoidDevRef"=w577) -> ("SolenoidDevRef"=w574:T2)  [unwired: 8 in, 1 out]
                n168 = call-poly <vilib>:"WPI_SolenoidSet.vi"("Value"=WPI_SolenoidValue."Off", "SolenoidDevRef"=w576) -> ("SolenoidDevRef"=w575:T2)  [unwired: 8 in, 1 out]
              }
            }
          }
        }
        frame #8 {
          # "Drive"
          n169 = for {
            N: 35 -> [_]
            shift-right: [w590] -> _
            shift-left: w584 -> [w589]
            n170 = Wait (ms)(milliseconds to wait=u32 10) -> ()  [unwired: 1 out]
            n171 = call-poly <vilib>:"WPI_RobotDriveArcadeDrive.vi"("Y axis value"=-0.6, "X axis value"=0.0, "RobotDriveDevRef"=w589) -> ("RobotDriveDevRef"=w590:T4)  [unwired: 6 in, 2 out]
          }
        }
      }
    }
  }
